vi "Set Frequency Filter [FRQ].vi"(7 "Micropulse # In":i32, 8 "error in (no error)":errorcluster, 9 "Smoothing":u16=1 caption="Smoothing (1-11)", 10 "Filter":T1, 11 "Test Number":u32) -> (0 "error out":errorcluster, 5 "Micropulse # Out":i32)   [LabVIEW 2026, in "MicroPulse_Driver.lvlib"]
doc: "For conventional channels this selects one of twelve frequency filters. The frequency filters are preferred probe centres frequencies or various broadband settings. For phased array channels this selects one of four filters. The third parameter defines for each test the level of smoothing on the rectified waveform.\n\nParameters:\n<Tn> : Test number. An integer value from 0 to the maximum number of tests (default maximum is 1279 tests).\nTn = 0 for all conventional tests. If the S extension is used it applies to all tests in the sweep number specified: 1-32, 0 = all sweeps.\n\n<Filter> (Conventional) :\n1 = 1 MHz Bandpass (0.75 - 1.7MHz 3dB Typ)\n2 = 2 MHz Bandpass (1.50 - 3.1MHz 3dB Typ)\n3 = 4 MHz Bandpass (2.60 - 5.5MHz 3dB Typ)\n4 = 5 MHz Bandpass (3.70 - 6.4MHz 3dB Typ)\n5 = 10 MHz Bandpass (8.20 - 12.0MHz 3dB Typ)\n6 = Broadband (2.50 - 18.0MHz)\n7 = Broadband (0.75 - 12.0MHz)\n8 = 0.5MHz Bandpass (0.30 - 0.8MHz 3dB Typ)\n9 = 5 MHz 2nd order TOFD (0.80 - 8.0MHz 3dB Typ)\n10 = 10 MHz 2nd order TOFD (3.00 - 15.0MHz 3dB Typ)\n11 = Broadband (3.00 - 22.0MHz)\n12 = Broadband (3.00 - 25.0MHz)\n\n<Filter> (Phased Array) :\n1 = 5.00 MHz to 10.0 MHz\n2 = 2.00 MHz to 10.0 MHz\n3 = 0.75 MHz to 5.00 MHz\n4 = 0.75 MHz to 20.0 MHz\n\n<Smoothing> :\nSets the level of smoothing on the rectified waveform for this test.\nAn integer value from 1 to 11\n\nExample : FRQ 0 2 7 : Sets 2 MHz filter and smoothing setting 7 to all conventional tests within the set NUM."
uses:
  MicroPulse_Driver.lvlib
  <instrlib>/MicroPulse/Public/Data/Datatypes/MP - frequency filter.ctl
  Private/MP-Registry Action-Enum.ctl
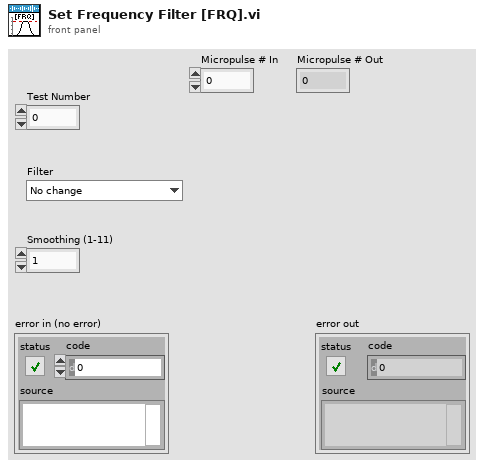
[diagram p1: front panel]
types:
  T1 = typedef "MicroPulse_Driver.lvlib/MP - frequency filter.ctl" = enum16{"No change", "1MHz Bandpass", "2MHz Bandpass", "4MHz Bandpass", "5MHz Bandpass", "10MHz Bandpass", "2.5-18MHz Broadband", "0.75-12MHz  Broadband", "0.5MHz Bandpass", "5MHz 2nd Order TOFD", "10MHz 2nd Order TOFD", "3.0-25MHz Broadband", "3.0-30MHz Broadband"}
  T2 = typedef "MicroPulse_Driver.lvlib/MP-Registry Action-Enum.ctl" = enum16{"Read", "Add Test", "Add Command", "Add Gate Command", "Add Encoder Command", "Clear Command  List", "Set Registry", "Set System Details", "Set DOF", "Set Velocity", "Disable Asynch Reads", "Enable Asynch Reads", "Add Connection", "Disconnect", "Shutdown"}
  T3 = typedef "MicroPulse_Driver.lvlib/MP-Registry Data-Cluster.ctl" = cluster{"Instrument Type":T4, "Serial #":u64, "Sample Frequency":T5, "dt (us)":dbl, "DOF":T6, "Material Velocity":dbl, "Asynch Reads":T7, "NUM of Tests":u32, "System Details":T8, "Gates":T10[], "Encoders":T17[], "CMD LUT":variant, "Command List":string}
  T4 = typedef "MicroPulse_Driver.lvlib/MP - instrument type.ctl" = enum16{"MicroPulse 5", "LT1", "LT2", "LTPA", "MPLT", "MicroPulse 6", "PipeScanner", "<MicroPulse>", "Micropulse 4", "Simulated Data"}
  T5 = typedef "MicroPulse_Driver.lvlib/MP - sample frequency.ctl" = enum16{"Use Default", "200MHz (LT2 only)", "100MHz", "50MHz", "25MHz", "10MHz"}
  T6 = typedef "MicroPulse_Driver.lvlib/MP - data output format.ctl" = enum16{"", "8-bit Mode", "10-bit Mode", "12-bit Mode", "16-bit Mode", "8-bit Log Mode", "12-bit Packed Mode"}
  T7 = typedef "MicroPulse_Driver.lvlib/MP - asynch read mode.ctl" = enum16{"Disabled", "Enabled"}
  T8 = typedef "MicroPulse_Driver.lvlib/MP - general system status.ctl" = cluster{"System Type":T4, "Serial No.":u64, "Channels":cluster{"Conv":u8, "PA":u16, "Extra":u32}, "Sample Frequency":cluster{"Default":u8, "Actual":u8}, "Software Versions":string, "Data Output Format":cluster{"Default":T6, "Actual":T6}, "Temperatures":cluster{"System":u8, "Processor":u8, "Slave Sys":u8, "Slave Proc":u8}, "Tx Buffer Size":u32, "System Error":string, "No. of Cards":u8, "DAC Gain":i16, "Uptimes":cluster{"since Power":u32, "since RSTS":u32, "since SRST":u32}, "Voltages":cluster{"Nominal":dbl, "Measured":dbl, "Difference":dbl}[], "Interface Cards":T9[]}
  T9 = typedef "MicroPulse_Driver.lvlib/MP - interface card status.ctl" = cluster{"Status":u8, "Map":u8, "Board - T":u8, "FPGA - T":u8, "PAIF Status":string, "Version":string}
  T10 = typedef "MicroPulse_Driver.lvlib/MP - Registry Gates.ctl" = cluster{"Display Gate":T11, "ETM Mode":T12, "Echo Gate":T13, "Insp Gates":T14[]}
  T11 = typedef "MicroPulse_Driver.lvlib/MP - display gate.ctl" = cluster{"Start":dbl, "Length":dbl}
  T12 = typedef "MicroPulse_Driver.lvlib/MP - echo gate mode.ctl" = enum16{"Echo Trigger OFF", "Echo Gate Display Mode", "Echo Trigger ON", "Multi Gate or FMC Mode", "Reserved", "PA - Echo Trigger ON"}
  T13 = typedef "MicroPulse_Driver.lvlib/MP - echo gate parameters.ctl" = cluster{"Start (us)":dbl, "Length (us)":dbl, "Threshold":u16, "Colour":u32}
  T14 = typedef "MicroPulse_Driver.lvlib/MP - multigate inspection gate parameters.ctl" = cluster{"Start (us)":dbl, "Length (us)":dbl, "Threshold":u16, "Enabled?":bool, "Max # Peaks":u16, "Hysteresis":T15, "Mode":T16, "Inverted?":bool, "Colour ":u32}
  T15 = typedef "MicroPulse_Driver.lvlib/MP - hysteresis level.ctl" = enum16{"None", "3dB", "6dB", "9dB", "12dB"}
  T16 = typedef "MicroPulse_Driver.lvlib/MP - multigate mode.ctl" = enum16{"1st Peak in Gate", "Largest Peak In Gate", "All Peaks In Gate", "1st Threshold Crossing"}
  T17 = typedef "MicroPulse_Driver.lvlib/MP - encoder settings.ctl" = cluster{"Encoder Type":T18, "Counts/mm":u32, "Enable Termination?":bool, "Multiplier":u32, "Backlash Period (s)":dbl, "Encoder Filter":u32}
  T18 = typedef "MicroPulse_Driver.lvlib/MP - encoder type.ctl" = enum16{"Quadrature", "Step/Direction"}
  T19 = typedef "MicroPulse_Driver.lvlib/TCP config.ctl" = cluster{"Connection ID":refnum<k5>, "IP address":string, "host port":u16, "OC timeout":i32, "Read timeout":i32, "Write timeout":i32}
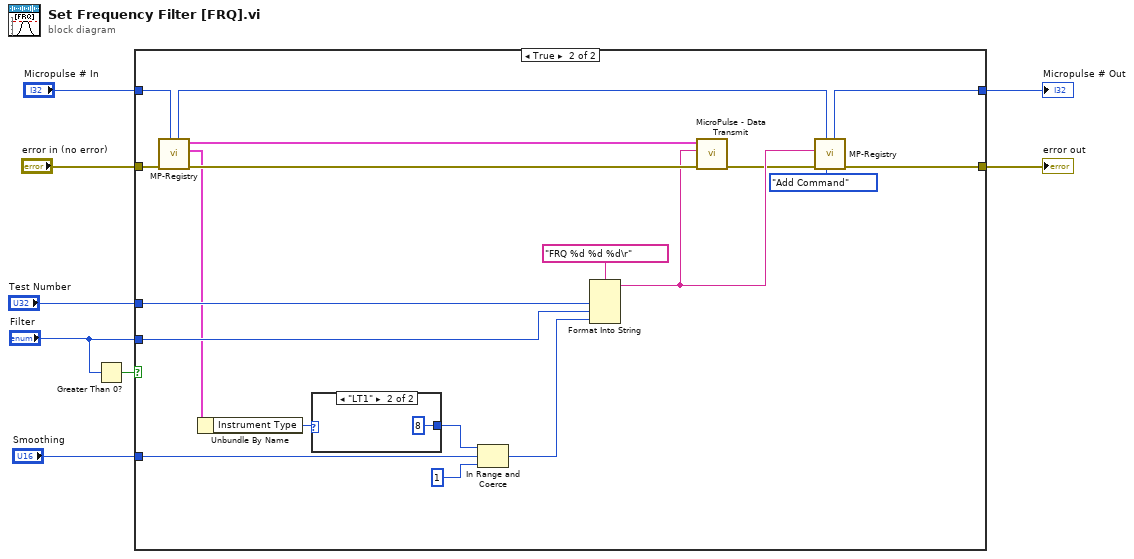
[diagram p0: block diagram]
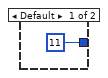
[diagram p3: hidden frame]
diagram:
  n1 = Greater Than 0?(x="Filter") -> (x > 0?=w3:bool)
  n2 = case shown="True" w3 {
    tunnel: "error in (no error)" -> [w9 w29]
    tunnel: "Micropulse # In" -> [w10 w28]
    tunnel: "Test Number" -> [_ w25]
    tunnel: "Smoothing" -> [_ w24]
    tunnel: [w9 w20] -> w5
    tunnel: [w10 w18] -> w4
    tunnel: "Filter" -> [_ w14]
    frame False {
    }
    frame True {
      n3 = call "MP-Registry.vi"("Micropulse # In"=w28, "error in (no error)"=w29) -> ("error out"=w27:errorcluster, "Micropulse Data"=w13:T3, "TCP config"=w26:T19, "Micropulse # Out"=w19:i32)  [unwired: 6 in]
      n4 = Unbundle By Name(w13) -> ("Instrument Type"=w12:T4)
      n5 = case shown="\"LT1\"" w12 {
        tunnel: [11 ("upper limit") 8 ("upper limit")] -> w11
        frame Default {
        }
        frame "LT1" {
        }
      }
      n6 = In Range and Coerce(upper limit=w11, x=w24, lower limit=1) -> (coerced(x)=w15:i32)  [unwired: 1 out]
      n7 = Format Into String(format string="FRQ %d %d %d\r", w25, w14, w15) -> (resulting string=w23:string)  [unwired: 2 in, 1 out]
      n8 = call "MicroPulse - Data Transmit.vi"("error in (no error)"=w27, "data"=w23, "TCP config"=w26) -> ("error out"=w21:errorcluster)  [unwired: 6 in, 2 out]
      n9 = call "MP-Registry.vi"("Action"=MP-Registry_Action-Enum."Add Command", "Micropulse # In"=w19, "error in (no error)"=w21, "Data in"=w23) -> ("error out"=w20:errorcluster, "Micropulse # Out"=w18:i32)  [unwired: 4 in, 2 out]
    }
  }
  "error out" <- w5
  "Micropulse # Out" <- w4
